vi "RSNRPZ Set Video Bandwidth.vi"(8 "error in (no error)":errorcluster, 9 "Bandwidth (0)":i32, 10 "Channel (1)":i32=1, 11 "VISA session":refnum<visa-resource-name> caption="VISA resource name") -> (0 "error out":errorcluster, 3 "dup VISA session":refnum<visa-resource-name> caption="VISA resource name")   [LabVIEW 2010]
doc: "This VI can be used to reduce the video bandwidth for the Trace and Statistics modes. As a result, trigger sensitivity is increased and the display noise reduced. To prevent signals from being corrupted, the selected video bandwidth should not be smaller than the RF bandwidth of the measurement signal. The \"FULL\" setting corresponds to a video bandwidth of at least 30 MHz if there is an associated frequency setting (SENSe:FREQuency command) greater than or equal to 500 MHz. If a frequency below 500 MHz is set and the video bandwidth is set to \"FULL\", the video bandwidth is automatically reduced to approx. 7.5 MHz.\nIf the video bandwidth is limited with the SENSe:BWIDth:VIDEo command, the sampling rate is also automatically reduced, i.e. the effective time resolution in the Trace mode is reduced accordingly. In the Statistics modes, the measurement time must be increased appropriately if the required sample size is to be maintained:\nVideo bandwidth Sampling rate Sampling interval\n\"Full\" 8e7 1/s 12.5 ns\n\"5 MHz\" 4e7 1/s 25 ns\n\"1.5 MHz\" 1e7 1/s 100 ns\n\"300 kHz\" 2.5e6 1/s 400 ns\n\n\n\n\n\n\n\n\nsets the video bandwidth according to a list of available bandwidths. The list can be obtained using VI rsnrpz_bandwidth_getBwList.\n\nRemote-control command(s):\nSENSe:BWIDth:VIDeo"
uses:
  rsnrpz_32.dll
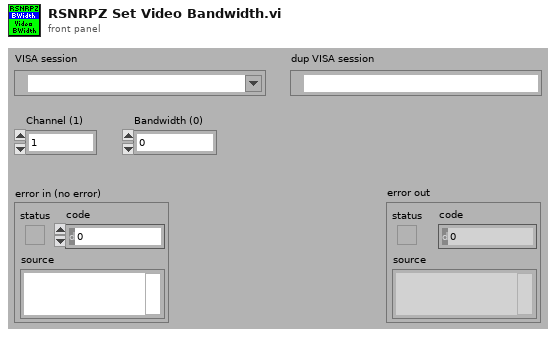
[diagram p1: front panel]
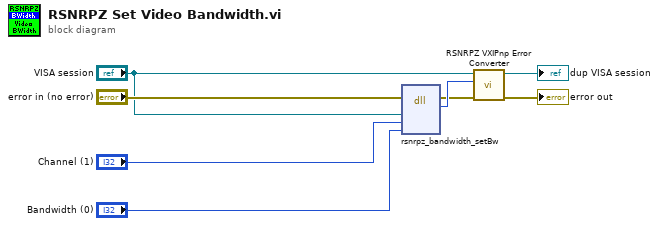
[diagram p0: block diagram]
diagram:
  n1 = dll-call lib="rsnrpz_32.dll" fn="rsnrpz_bandwidth_setBw"(error in="error in (no error)", "Instrument Handle"="VISA session", "Channel"="Channel (1)", "Bandwidth"="Bandwidth (0)") -> (error out=w5:errorcluster, "Status"=w8:i32)  [unwired: 5 in, 1 out]
  n2 = call <instrlib>:"RSNRPZ VXIPnp Error Converter.vi"("error in"=w5, "VXIPnp error code"=w8, "VISA session"="VISA session") -> ("error out"=→"error out":errorcluster, "dup VISA session"=→"dup VISA session":refnum<visa-resource-name>)  [unwired: 7 in]
